vi "Wrap Non-Object Values.vi"(10 "<JSON> in":string) -> (2 "<JSON> out":string)   [LabVIEW 2017, in "JSON Serializable Serializer.lvclass"]
doc: "Wraps non-object values in a custom JSON object with key \"$data\". Does nothing if the provided JSON is already an object or not a JSON value.\n\n<B>Example</B>\n[1,2,3] => {\"$data\",[1,2,3]}"
uses:
  JSON Serializable Serializer.lvclass
  <vilib>/JDP Science/JSONtext/JSONtext.lvlib
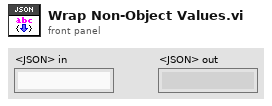
[diagram p1: front panel]
types:
  T1 = typedef "JSONtext.lvlib/JSON Value Type.ctl" = enum16{"Not a JSON Value", "JSON Object", "JSON Array", "String", "Number", "true", "false", "null"}
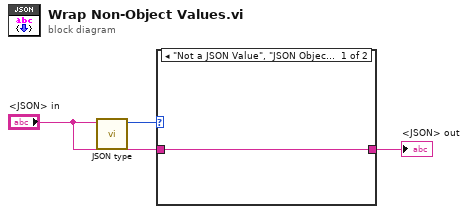
[diagram p0: block diagram]
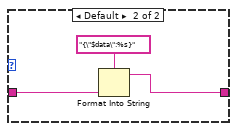
[diagram p2: hidden frame]
diagram:
  n1 = call <vilib>:"JSON type.vi"("JSON"="<JSON> in") -> ("JSON Value Type"=w3:T1)  [unwired: 9 in, 1 out]
  n2 = case shown="\"Not a JSON Value\", \"JSON Object\"" w3 {
    tunnel: "<JSON> in" -> [w4 w6]
    tunnel: [w4 w5] -> w1
    frame "Not a JSON Value", "JSON Object" {
    }
    frame Default {
      n3 = Format Into String(format string="{\"$data\":%s}", w6) -> (resulting string=w5:string)  [unwired: 2 in, 1 out]
    }
  }
  "<JSON> out" <- w1
